vi "Calculate Button Repeats.vi"(11 "Previous Button State":T1=enum."Pressed") -> (3 "New Buton State":T1=enum."Pressed")   [LabVIEW 2021, in "Control State.lvclass"]
uses:
  Control State.lvclass
  Button State.ctl
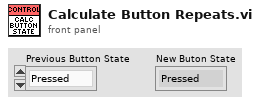
[diagram p1: front panel]
types:
  T1 = typedef "Control State.lvclass/Button State.ctl" = enum16{"Undefined", "Pressed", "Released", "Held", "Not Held"}
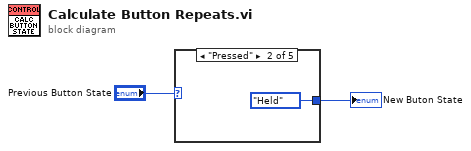
[diagram p0: block diagram]
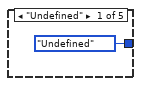
[diagram p2: hidden frame]
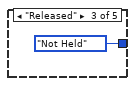
[diagram p3: hidden frame]
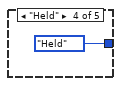
[diagram p4: hidden frame]
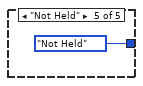
[diagram p5: hidden frame]
diagram:
  n1 = case shown="\"Pressed\"" "Previous Button State" {
    tunnel: [Button_State."Undefined" ("Primary Weapon") Button_State."Held" ("Primary Weapon") Button_State."Not Held" ("Primary Weapon") Button_State."Held" ("Primary Weapon") Button_State."Not Held" ("Primary Weapon")] -> w2
    frame "Undefined" {
    }
    frame "Pressed" {
    }
    frame "Released" {
    }
    frame "Held" {
    }
    frame "Not Held" {
    }
  }
  "New Buton State" <- w2
